vi "calculate score.vi"(9 "Game Parameters":T3, 10 "loop count":i32, 11 "Arrays and Heights":T1={"Score Array"=[], "Lowest high score"=0.0, "Score"=0.0, "Ceiling"=0.0, "Floor"=0.0, "Ceiling Array"=[], "Floor array"=[], "Helicopter height"=0.0, "Helicopter array"=[], "Fuel"=300.0, "Fuel array"=[], "fuel counter"=0, "obstacle counter"=0, "Obstacle array"=[], "helicopter v_0"=0.0, "helicopter a_0"=0.0, "Obstacle height"=300.0}) -> (2 "Score":dbl, 3 "Arrays and Heights":T1={"Score Array"=[], "Lowest high score"=0.0, "Score"=0.0, "Ceiling"=0.0, "Floor"=0.0, "Ceiling Array"=[], "Floor array"=[], "Helicopter height"=0.0, "Helicopter array"=[], "Fuel"=300.0, "Fuel array"=[], "fuel counter"=0, "obstacle counter"=0, "Obstacle array"=[], "helicopter v_0"=0.0, "helicopter a_0"=0.0, "Obstacle height"=300.0})   [LabVIEW 2017]
uses:
  controls/game parameters.ctl
  controls/arrays and heights.ctl
  controls/scores.ctl
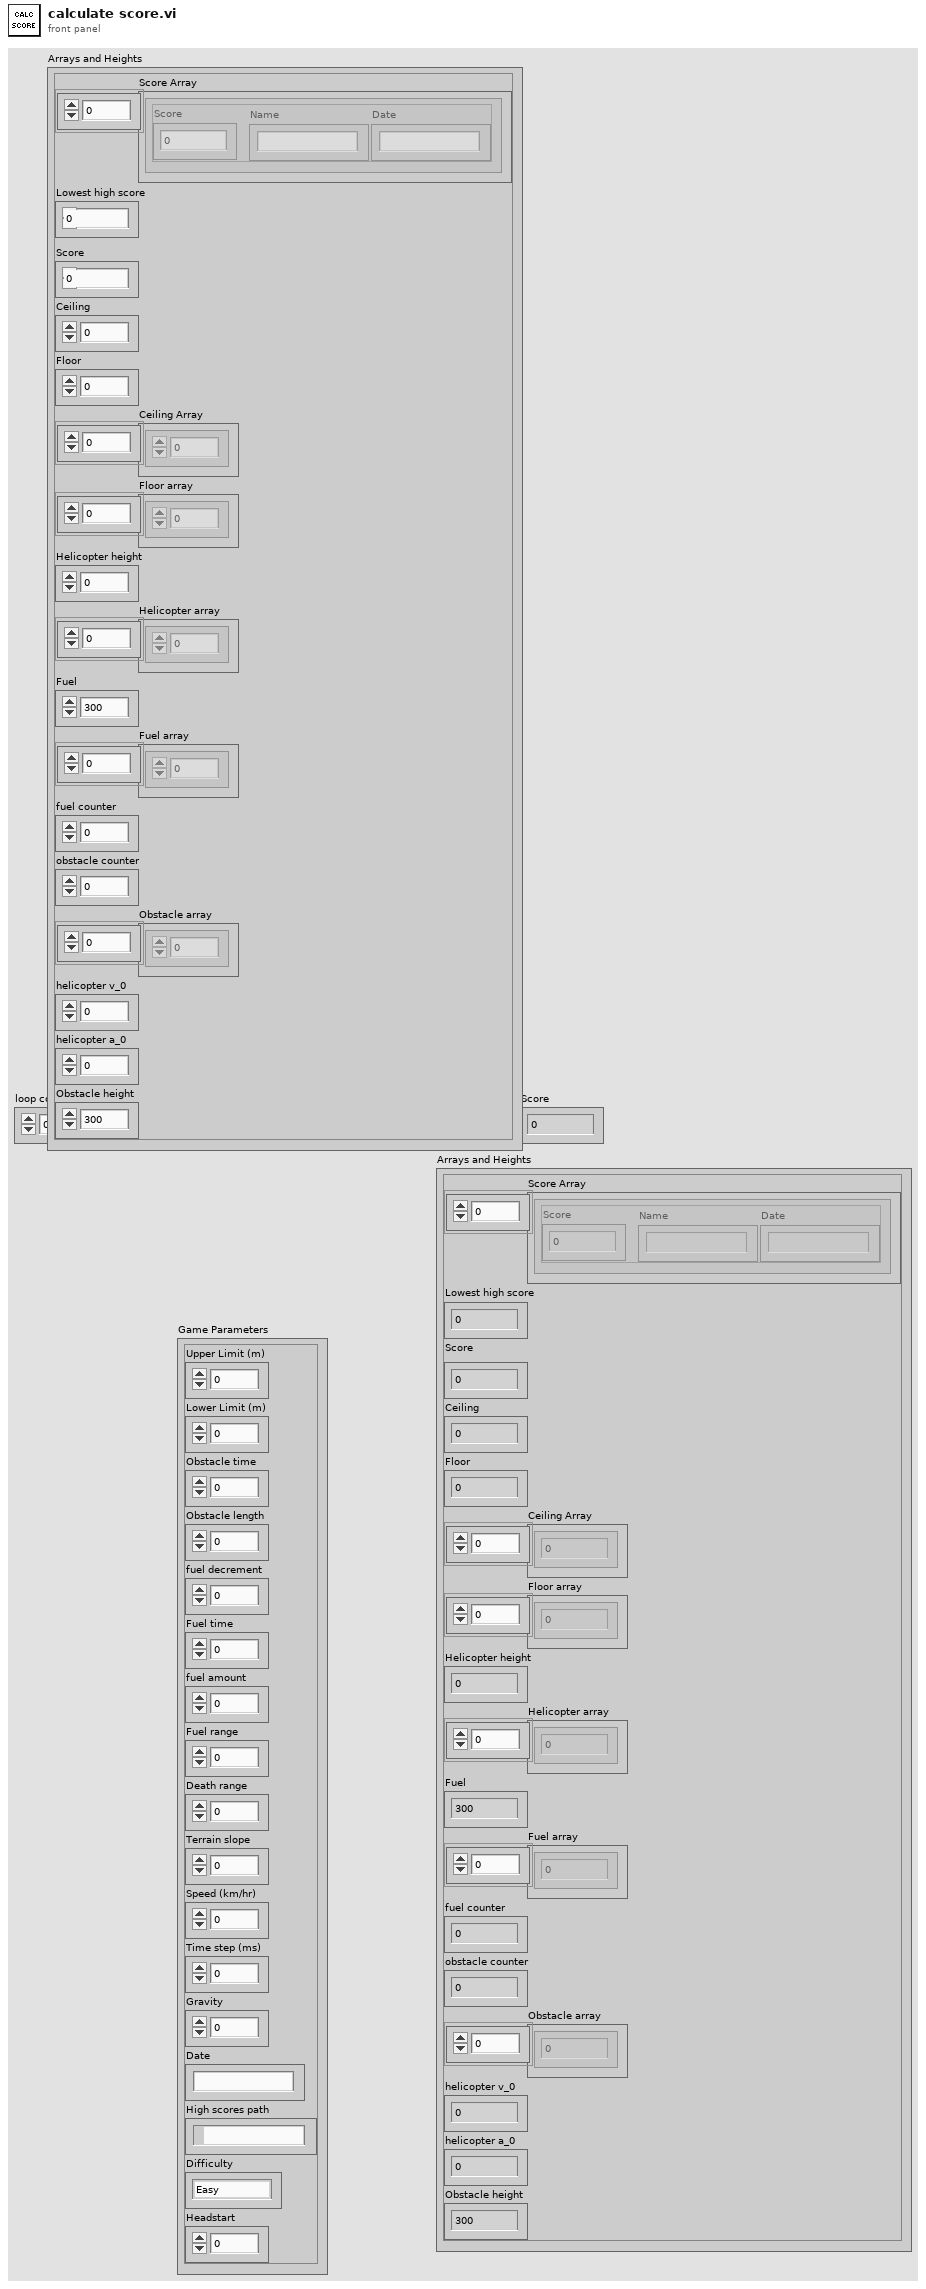
[diagram p1: front panel]
types:
  T1 = typedef "arrays and heights.ctl" = cluster{"Score Array":T2[], "Lowest high score":dbl, "Score":dbl, "Ceiling":dbl, "Floor":dbl, "Ceiling Array":dbl[], "Floor array":dbl[], "Helicopter height":dbl, "Helicopter array":dbl[], "Fuel":dbl, "Fuel array":dbl[], "fuel counter":i32, "obstacle counter":i32, "Obstacle array":dbl[], "helicopter v_0":dbl, "helicopter a_0":dbl, "Obstacle height":dbl}
  T2 = typedef "scores.ctl" = cluster{"Score":dbl, "Name":string, "Date":string}
  T3 = typedef "game parameters.ctl" = cluster{"Upper Limit (m)":dbl, "Lower Limit (m)":dbl, "Obstacle time":dbl, "Obstacle length":dbl, "fuel decrement":dbl, "Fuel time":dbl, "fuel amount":dbl, "Fuel range":i32, "Death range":i32, "Terrain slope":dbl, "Speed (km/hr)":dbl, "Time step (ms)":u32, "Gravity":dbl, "Date":string, "High scores path":path, "Difficulty":enum16{"Easy", "Normal", "Hard"}, "Headstart":u32}
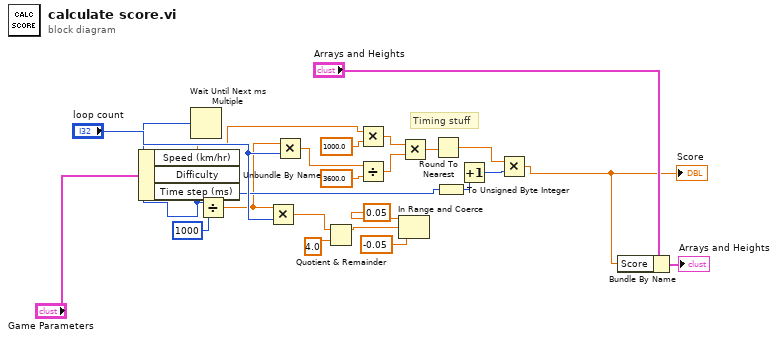
[diagram p0: block diagram]
diagram:
  # "Timing stuff"
  n1 = Unbundle By Name("Game Parameters") -> ("Speed (km/hr)"=w4:dbl, "Difficulty"=w21:enum16{"Easy", "Normal", "Hard"}, "Time step (ms)"=w23:u32)
  n2 = Wait Until Next ms Multiple(millisecond multiple=w23) -> ()  [unwired: 1 out]
  n3 = Divide(x=w23, y=u32 1000) -> (x/y=w16:dbl)
  n4 = Multiply(x=w16, y="loop count") -> (x*y=w11:dbl)
  n5 = Multiply(x=w16, y="loop count") -> (x*y=w17:dbl)
  n6 = Quotient & Remainder(x=w11, y=4.0) -> (x-y*floor(x/y)=w13:dbl)  [unwired: 1 out]
  n7 = Multiply(x=w4, y=1000.0) -> (x*y=w8:dbl)
  n8 = Divide(x=w17, y=3600.0) -> (x/y=w7:dbl)
  n9 = In Range and Coerce(upper limit=0.05, x=w13, lower limit=-0.05) -> ()  [unwired: 2 out]
  n10 = Multiply(x=w8, y=w7) -> (x*y=w9:dbl)
  n11 = Round To Nearest(number=w9) -> (nearest integer value=w18:dbl)
  n12 = To Unsigned Byte Integer(number=w21) -> (unsigned 8bit integer=w20:u8)
  n13 = Increment(x=w20) -> (x+1=w19:u8)
  n14 = Multiply(x=w18, y=w19) -> (x*y=w2:dbl)
  "Score" <- w2
  n15 = Bundle By Name(cluster="Arrays and Heights", "Score"=w2) -> (→"Arrays and Heights":T1)
